vi "Set Test Node Tiles Info.vi"(8 "error in (no error)":errorcluster, 10 "Test Node Tiles Info":string[][](array[string]), 11 "Abstract Test Node Tiles Info Msg in":refnum<class "Abstract Test Node Tiles Info Msg.lvclass">) -> (0 "error out":errorcluster, 3 "Abstract Test Node Tiles Info Msg out":refnum<class "Abstract Test Node Tiles Info Msg.lvclass">)   [LabVIEW 2013, in "Test Node Model.lvlib" / "Abstract Test Node Tiles Info Msg.lvclass"]
uses:
  Abstract Test Node Tiles Info Msg.lvclass
  Abstract Test Node Tiles Info Msg.lvclass/Abstract Test Node Tiles Info Msg.ctl
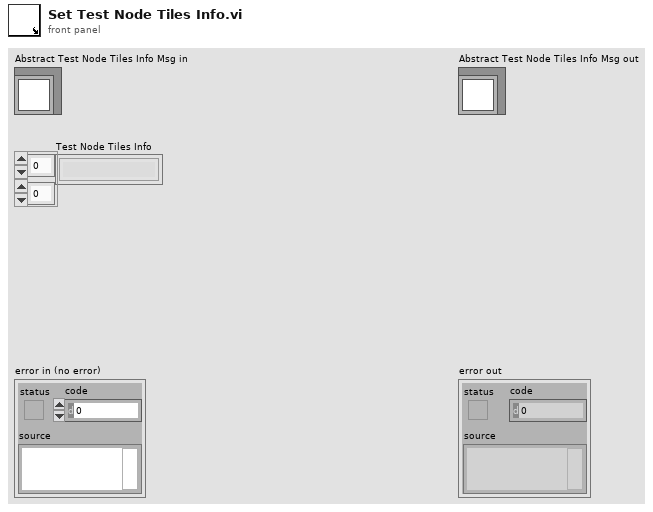
[diagram p1: front panel]
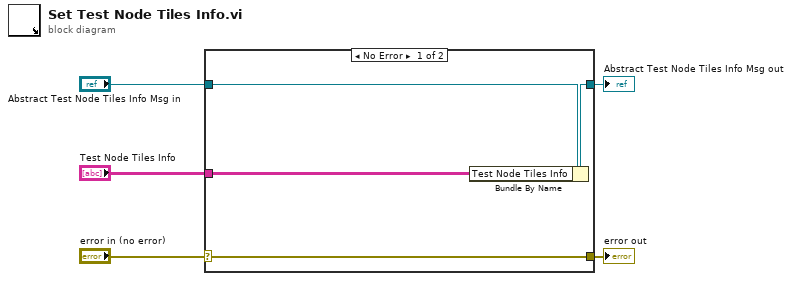
[diagram p0: block diagram]
diagram:
  n1 = case shown="No Error" "error in (no error)" {
    selector: "error in (no error)" -> [w9 w10]
    tunnel: [w9 w10] -> w4
    tunnel: [w7 w11] -> w2
    tunnel: "Abstract Test Node Tiles Info Msg in" -> [w8 w11]
    tunnel: "Test Node Tiles Info" -> [w6 _]
    frame No Error {
      n2 = Bundle By Name(cluster=w8, "Test Node Tiles Info"=w6) -> (w7:refnum<class "Abstract Test Node Tiles Info Msg.lvclass">)
    }
    frame Error {
    }
  }
  "error out" <- w4
  "Abstract Test Node Tiles Info Msg out" <- w2
